vi "Dashboard Main.vi"() -> ()   [LabVIEW 2013]
uses:
  <vilib>/event_ctls.llb/eventvkey.ctl
  <vilib>/Utility/config.llb/NI_LVConfig.lvlib
  <vilib>/Utility/config.llb/Write Key (I32).vi
  <vilib>/Rock Robotics/WPI/Dashboard/WPI_DashboardLogging Global.vi
  <vilib>/Utility/config.llb/Write Key (String).vi
panel:
  out "Image Message":string="Timeout in Camera Communications"
  in  "Rec Mode":enum32{"Stop", "Record", "Playback"}(radio)
  in  "Dashboard Tab":T1(tab)
  out "Left Encoder Distance":dbl
  out "Left Encoder Revolutions":dbl
  out "Left Encoder Agnle":dbl
  out "Right Encoder Distance":dbl
  out "Right Encoder Revolutions":dbl
  out "Right Encoder Agnle":dbl
  out "Slow Drive":bool
  out "Can Shoot":bool
  out "Camera Sonar":dbl
  out "Rear Sonar":dbl
  out "Front Left Sonar":dbl
  out "Front Right Sonar":dbl
  out "Ball in Cannon":bool
  out "Cannon Angle":dbl(knob) scale=0.0..360.0
  out "InTake Angle":dbl(knob) scale=0.0..360.0
  in  "Camera Settings":T2={"Frame Rate"=30, "Compression"=30, "Size"=1} {"Frame Rate" scale=1.0..30.0; "Size" items=["640x480", "320x240", "160x120"]}
  out "MotorSliders R":cluster{"MotorSlide1":dbl, "MotorSlide2":dbl} {"MotorSlide2" scale=-1.0..1.0 scale format="%#_2e"; "MotorSlide1" scale=-1.0..1.0 scale format="%#_2e"}
  out "MotorChart R":cluster{"Numeric":dbl, "Numeric":dbl}(graph)
  out "MotorSliders L":T3 {"MotorSlide4 2" scale=0.0..14.0 scale format="%#_2e"; "MotorSlide2" scale=-1.0..1.0 scale format="%#_2e"; "MotorSlide1" scale=-1.0..1.0 scale format="%#_2e"}
  out "MotorChart L":T4(graph)
  out "JS1 Z":dbl(slide) scale=-1.0..1.0 scale format="%#_2e"
  out "Joystick 1":cluster{"X":dbl, "Y":dbl}[](graph)
  out "JS Buttons 1":T5
  out "JS2 Z":dbl(slide) scale=-1.0..1.0 scale format="%#_2e"
  out "Joystick 2":cluster{"X":dbl, "Y":dbl}[](graph)
  out "JS Buttons 2":T5
  out "Mode":T6(ring)=enum."Auto Disabled"
  out "Camera IP":string
  in  "DB Camera Config":bool
  out "fps":dbl format="%#.1g"
  out "Mbps":dbl format="%#.1g"
  out "Mbps 2":bool
  out "Joystick 3":cluster{"X":dbl, "Y":dbl}[](graph)
  out "JS Buttons 3":T5
  out "JS1 Z 2":dbl(slide) scale=-1.0..1.0 scale format="%#_2e"
  out "Joystick 4":cluster{"X":dbl, "Y":dbl}[](graph)
  out "JS2 Z 2":dbl(slide) scale=-1.0..1.0 scale format="%#_2e"
  out "JS Buttons 4":T5
  in  "Read From Dashboard":bool
  in  "Operator":T7 {"Left Y 2" scale=-1.0..1.0; "Left X 2" scale=-1.0..1.0; "Right Y 2" scale=-1.0..1.0; "Right X 2" scale=-1.0..1.0}
  in  "Drive":T8 {"Left Y" scale=-1.0..1.0; "Left X" scale=-1.0..1.0; "Right Y" scale=-1.0..1.0; "Right X" scale=-1.0..1.0}
  in  "Test Slider":dbl(slide) scale=0.0..100.0 scale format="%#_3g"
  in  "On/Off":bool caption="Solenoid"
  in  "Test Name":u16(ring) items=["Select the test to run...", "Example Test", "-------------------------------", "List of tests is built in robot code.", "Replace with your own automated tests."]
  in  "Test Tree":string(tree)
  in  "Motor":cluster{"Value":dbl, "Enable":bool} {"Value" scale=-1.0..1.0 scale format="%#_3g"}
  out "Progress":T9 {"Test Progress" scale=0.0..100.0}
  in  "Rev/Fwd":cluster{"Forward":bool, "Reverse":bool}
  in  "Test Ring":u16(ring) items=["Auto", "Fixed indoor", "Fixed outdoor 1", "Fixed outdoor 2", "Fixed fluorescent 1", "Fixed fluorescent 2", "Hold current"]
  in  "Listbox":i32(listbox)
  out "Tree":string(tree)
  out "Camera Image":T10(plugin-control)
  in  "Enable":bool
  # "Operation"
  # "Left"
  # "Right"
  # "Left"
  # "Front"
  # "Right"
  # "Battery"
  # "Operation"
  # "Drive"
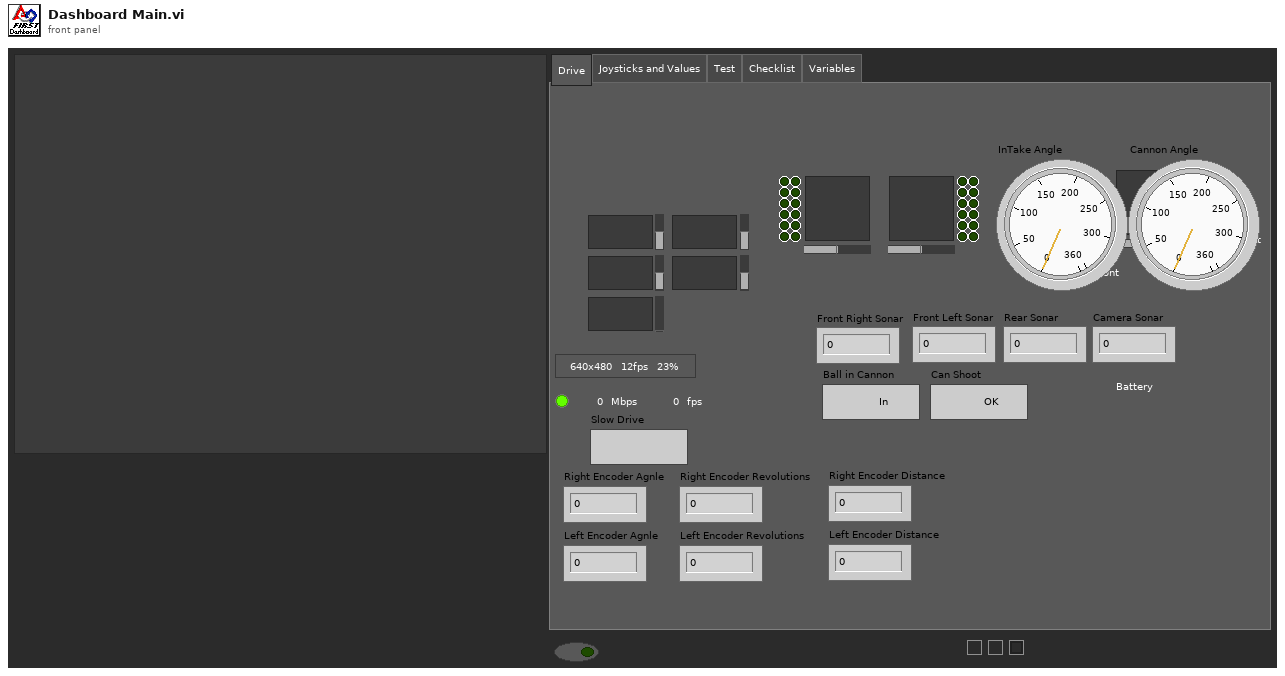
[diagram p1: front panel]
types:
  T1 = enum32{"Drive", "Joysticks and Values", "Test", "Checklist", "Variables"}
  T2 = cluster{"Frame Rate":i32, "Compression":i32, "Size":u16}
  T3 = cluster{"MotorSlide1":dbl, "MotorSlide2":dbl, "MotorSlide4 2":dbl}
  T4 = cluster{"Numeric":dbl, "Numeric":dbl, "Battery":sgl}
  T5 = cluster{bool, bool, bool, bool, bool, bool, bool, bool, bool, bool, bool, bool}
  T6 = enum8{"Tele-Op Disabled", "Tele-Op Enabled", "Auto Disabled", "Auto Enabled", "Test Disabled", "Test Enabled", ""}
  T7 = cluster{"Right X 2":dbl, "Right Y 2":dbl, "Left X 2":dbl, "Left Y 2":dbl, "Arrows 2":dbl, "Left Stick Touch  2":bool, "Right Stick Touch 2":bool, "Left Button  2":bool, "Right Button 2":bool, "L+R Throttles 2":dbl, "Center Right 2":bool, "Center Left 2":bool, "X 2":bool, "A 2":bool, "B 2":bool, "Y 2":bool}
  T8 = cluster{"Right X":dbl, "Right Y":dbl, "Left X":dbl, "Left Y":dbl, "Arrows":dbl, "Left Stick Touch ":bool, "Right Stick Touch":bool, "Left Button ":bool, "Right Button":bool, "L+R Throttles":dbl, "Center Right":bool, "Center Left":bool, "X":bool, "A":bool, "B":bool, "Y":bool}
  T9 = cluster{"Test Progress":u8, "Test Progress Text":string}
  T10 = typedef "IMAQ Image.ctl" = refnum<image>
  T11 = enum32{"Drive", "Operation", "Auto", "Test", "Checklist", "Variables"}
  T12 = typedef "Image Type" = u32
  T13 = cluster{"[0]":void, "[1]":void, "[2]":void, "[3]":void, "[4]":void, "[5]":void, "[6]":void, "[7]":void, "[8]":void}
  T14 = cluster{"Digital Inputs":bool[], "Digital Outputs":bool[]}
  T15 = cluster{"Competition mode":bool, "Robot Link":bool, "Autonomous":bool, "Enabled":bool, "E-Stop":bool, "Simulated":bool, "TestMode":bool, "Docked Window":bool}
  T16 = cluster{"Boolean Array[0]":bool, "Boolean Array[1]":bool, "Boolean Array[2]":bool, "Boolean Array[3]":bool, "Boolean Array[4]":bool, "Boolean Array[5]":bool, "Boolean Array[6]":bool, "Boolean Array[7]":bool, "Boolean Array[8]":bool, "Boolean Array[9]":bool, "Boolean Array[10]":bool, "Boolean Array[11]":bool}
  T17 = typedef "NI_LVConfig.lvlib/Config Data RefNum.ctl" = refnum<k1>
  T18 = typedef "eventvkey.ctl" = enum16{"ASCII", "Enter", "Return", "Shift", "Ctrl", "Alt", "Cmd", "Opt", "Caps", "NumLock", "Clear", "Break", "Up", "Down", "Left", "Right", "Insert", "Delete", "Home", "End", "PageUp", "PageDown", "Escape", "Help", "Pause", "ScrollLock", "F1", "F2", "F3", "F4", "F5", "F6", "F7", "F8", "F9", "F10", "F11", "F12", "F13", "F14", "F15", "F16", "F17", "F18", "F19", "F20", "F21", "F22", "F23", "F24", "Play", "VolumeUp", "VolumeDown", "Mute", "Two Byte Char"}
  T19 = cluster{"Image Size":bool, "Image Type":bool, "Pixel Value":bool, "ROI Information":bool, "Zoom Factor":bool}
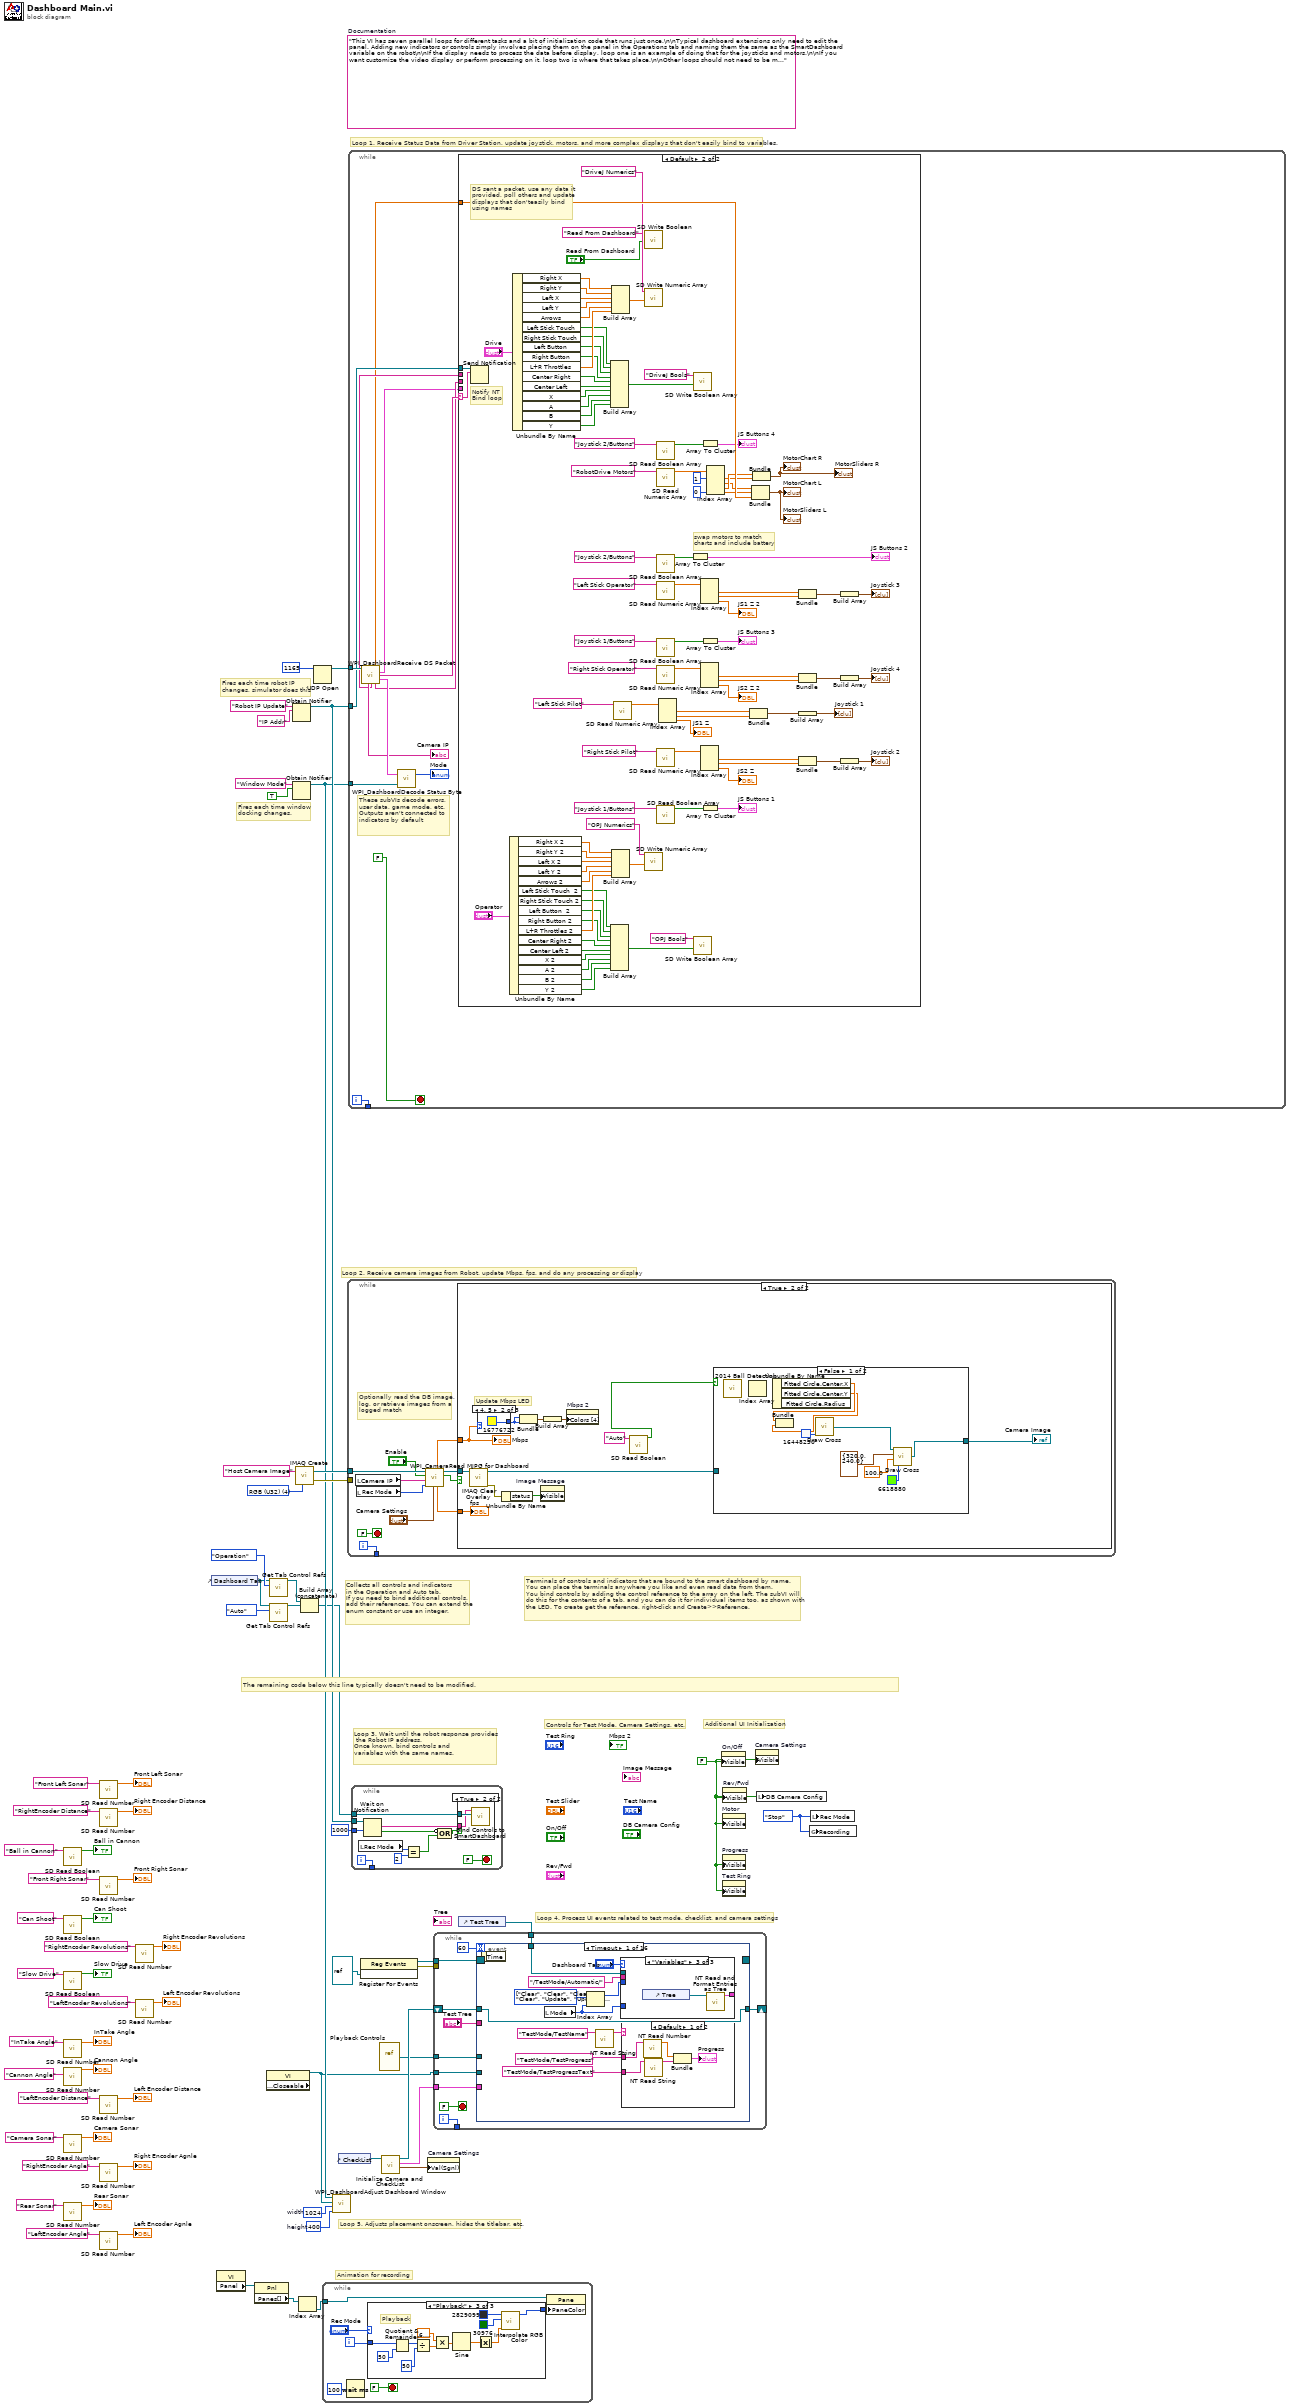
[diagram p0: block diagram]
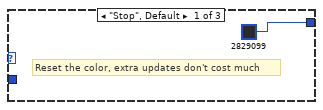
[diagram p2: hidden frame]
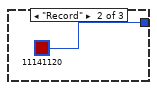
[diagram p3: hidden frame]
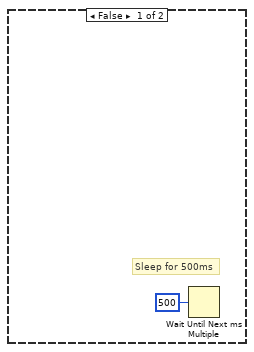
[diagram p5: hidden frame]
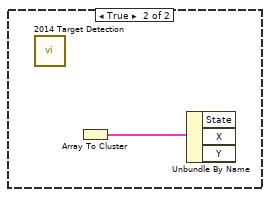
[diagram p6: hidden frame]
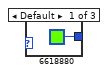
[diagram p7: hidden frame]
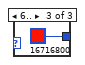
[diagram p8: hidden frame]
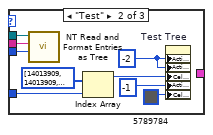
[diagram p10: hidden frame]
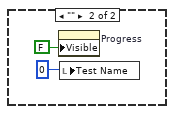
[diagram p11: hidden frame]
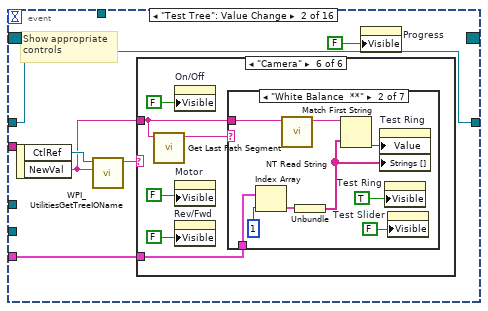
[diagram p12: hidden frame]
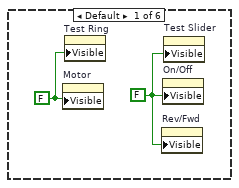
[diagram p13: hidden frame]
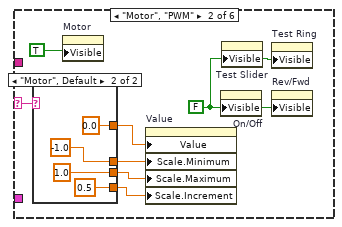
[diagram p14: hidden frame]
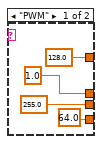
[diagram p15: hidden frame]
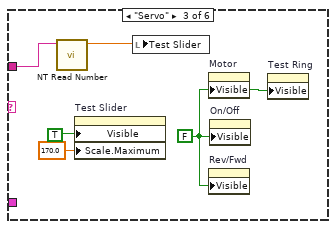
[diagram p16: hidden frame]
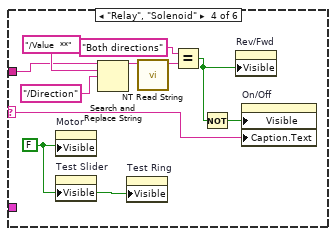
[diagram p17: hidden frame]
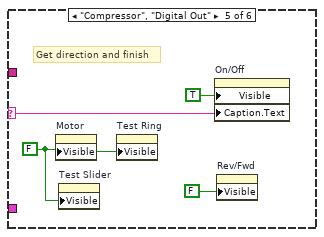
[diagram p18: hidden frame]
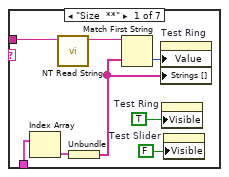
[diagram p19: hidden frame]
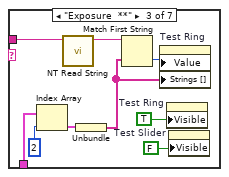
[diagram p20: hidden frame]
diagram:
  w38 = enum32{"Stop", "Record", "Playback"}."Stop" ("Rec Mode")
  w41 = 400  # height
  w42 = 1024  # width
  w55 = FALSE ("Visible")
  (unwired) "This VI has seven parallel loops for different tasks and a bit of initialization code that runs just once.\n\nTypical dashboard extensions only need to edit the panel. Adding new indicators or controls simply involves placing them on the panel in the Operations tab and naming them the same as the SmartDashboard variable on the robot\n\nIf the display needs to process the data before display, loop one is an example of doing that for the joysticks and motors.\n\nIf you want customize the video display or perform processing on it, loop two is where that takes place.\n\nOther loops should not need to be modified. They are pretty standard, and document the task they perform."  # Documentation
  w65 = T12 4 items=["Grayscale (U8)", "Grayscale (I16)", "Grayscale (SGL)", "Complex (CSG)", "RGB (U32)", "HSL (U32)", "RGB (U64)"] ("Image Type")
  # "Controls for Test Mode, Camera Settings, etc."
  # "Additional UI Initialization"
  # "Animation for recording"
  # "Fires each time robot IP\nchanges, simulator does this"
  # "Fires each time window\ndocking changes."
  # "Collects all controls and indicators\nin the Operation and Auto tab.\nIf you need to bind additional controls,\nadd their references. You can extend the\nenum constant or use an integer."
  # "The remaining code below this line typically doesn't need to be modified."
  # "Loop 4. Process UI events related to test mode, checklist, and camera settings"
  # "Terminals of controls and indicators that are bound to the smart dashboard by name.\nYou can place the terminals anywhere you like and even read data from them.\nYou bind controls by adding the control reference to the array on the left. The subVI will\ndo this for the contents of a tab, and you can do it for individual items too, as shown with\nthe LED. To create get the reference, right-click and Create>>Reference."
  # "Loop 3. Wait until the robot response provides\n the Robot IP address.\nOnce known, bind controls and\nvariables with the same names."
  # "Loop 5. Adjusts placement onscreen, hides the titlebar, etc."
  # "Loop 1. Receive Status Data from Driver Station, update joystick, motors, and more complex displays that don't easily bind to variables."
  # "Loop 2. Receive camera images from Robot, update Mbps, fps, and do any processing or display"
  n1 = call <vilib>:"SD Read Boolean.vi"("Name"="Ball in Cannon") -> ("Boolean"=→"Ball in Cannon":bool)  [unwired: 8 in, 2 out]
  n2 = call <vilib>:"SD Read Boolean.vi"("Name"="Can Shoot") -> ("Boolean"=→"Can Shoot":bool)  [unwired: 8 in, 2 out]
  n3 = call <vilib>:"SD Read Boolean.vi"("Name"="Slow Drive") -> ("Boolean"=→"Slow Drive":bool)  [unwired: 8 in, 2 out]
  n4 = call <vilib>:"SD Read Number.vi"("Name"="InTake Angle") -> ("Numeric"=→"InTake Angle":dbl)  [unwired: 8 in, 2 out]
  n5 = call <vilib>:"SD Read Number.vi"("Table Prefix"="Cannon Angle" ("Name")) -> ("Numeric"=→"Cannon Angle":dbl)  [unwired: 8 in, 2 out]
  n6 = call <vilib>:"SD Read Number.vi"("Name"="Camera Sonar") -> ("Numeric"=→"Camera Sonar":dbl)  [unwired: 8 in, 2 out]
  n7 = call <vilib>:"SD Read Number.vi"("Name"="Rear Sonar") -> ("Numeric"=→"Rear Sonar":dbl)  [unwired: 8 in, 2 out]
  n8 = call <vilib>:"SD Read Number.vi"("Name"="Front Left Sonar") -> ("Numeric"=→"Front Left Sonar":dbl)  [unwired: 8 in, 2 out]
  n9 = call <vilib>:"SD Read Number.vi"("Name"="RightEncoder Distance") -> ("Numeric"=→"Right Encoder Distance":dbl)  [unwired: 8 in, 2 out]
  n10 = call <vilib>:"SD Read Number.vi"("Name"="Front Right Sonar") -> ("Numeric"=→"Front Right Sonar":dbl)  [unwired: 8 in, 2 out]
  n11 = call <vilib>:"SD Read Number.vi"("Name"="LeftEncoder Distance") -> ("Numeric"=→"Left Encoder Distance":dbl)  [unwired: 8 in, 2 out]
  n12 = call <vilib>:"SD Read Number.vi"("Name"="RightEncoder Angle") -> ("Numeric"=→"Right Encoder Agnle":dbl)  [unwired: 8 in, 2 out]
  n13 = call <vilib>:"SD Read Number.vi"("Name"="LeftEncoder Angle") -> ("Numeric"=→"Left Encoder Agnle":dbl)  [unwired: 8 in, 2 out]
  n14 = call <vilib>:"SD Read Number.vi"("Name"="RightEncoder Revolutions") -> ("Numeric"=→"Right Encoder Revolutions":dbl)  [unwired: 8 in, 2 out]
  n15 = call <vilib>:"SD Read Number.vi"("Name"="LeftEncoder Revolutions") -> ("Numeric"=→"Left Encoder Revolutions":dbl)  [unwired: 8 in, 2 out]
  n16 = control-ref of="Dashboard Tab"() -> (w36:refnum<vi>)
  n17 = property class="VI"() -> ("Panel"=w49:refnum<vi>)  [unwired: 2 in, 2 out]
  n18 = property class="Pnl"(reference=w49) -> ("Panes[]"=w50:refnum<vi>[])  [unwired: 1 in, 2 out]
  n19 = property class="VI" props=["Front Panel.Closeable"]() -> (reference out=w37:refnum<vi>)  [unwired: 2 in, 2 out]
  n20 = call <vilib>:"Get Tab Control Refs.vi"("Page Index"=T11."Operation" ("Dashboard Tab"), "TabControl in"=w36) -> ("ControlsOnPage"=w34:refnum<vi>[])  [unwired: 9 in]
  n21 = call <vilib>:"Get Tab Control Refs.vi"("Page Index"=T11."Auto" ("Dashboard Tab"), "TabControl in"=w36) -> ("ControlsOnPage"=w35:refnum<vi>[])  [unwired: 9 in]
  n22 = Obtain Notifier(name (unnamed)="Robot IP Update", notification data type="IP Addr" ("name (unnamed)")) -> (notifier out=w59:refnum<notifier>)  [unwired: 2 in, 2 out]
  n23 = Obtain Notifier(name (unnamed)="Window Mode", notification data type=TRUE) -> (notifier out=w40:refnum<notifier>)  [unwired: 2 in, 2 out]
  n24 = call "IMAQ Create"("Image Name"="Host Camera Image", "Image Type"=w65) -> ("New Image"=w63:T10, "error out"=w62:errorcluster)  [unwired: 2 in, 1 out]
  n25 = Index Array(array=w50) -> (element=w48:refnum<vi>)  [unwired: 1 in]
  n26 = Build Array (concatenate)(w34, w35) -> (w33:refnum<vi>[], w31:refnum<vi>[])
  n27 = UDP Open(11:u16 1165 ("port")) -> (port=w66:refnum<k16>)  [unwired: 2 in, 4 out]
  n28 = while {
    tunnel: w48 -> [w69]
    i -> [w72]
    stop <- FALSE stop-if-true
    n29 = Wait (ms)(milliseconds to wait=u32 100) -> ()  [unwired: 1 out]
    n30 = case shown="\"Playback\"" "Rec Mode" {
      tunnel: w72 -> [_ _ w87]
      tunnel: [u32 2829099 ("Base Color") u32 11141120 ("Target Color") w76] -> w68
      frame "Stop", Default {
        # "Reset the color, extra updates don't cost much"
      }
      frame "Record" {
      }
      frame "Playback" {
        # "Playback"
        n31 = Quotient & Remainder(x=w87, y=u32 50 ("milliseconds to wait")) -> (x-y*floor(x/y)=w83:u32)  [unwired: 1 out]
        n32 = Divide(x=w83, y=u32 50 ("milliseconds to wait")) -> (x/y=w80:dbl)
        n33 = Multiply(x=6.283185307179586, y=w80) -> (x*y=w85:dbl)
        n34 = Sine(x=w85) -> (sin(x)=w84:dbl)
        n35 = Absolute Value(x=w84) -> (abs(x)=w77:dbl)
        n36 = call "Interpolate RGB Color.vi"("Proportion"=w77, "Target Color"=u32 30976, "Base Color"=u32 2829099) -> ("Result Color"=w76:u32)  [unwired: 8 in]
      }
    }
    n37 = property class="Pane"(reference=w69, "PaneColor"=w68) -> ()  [unwired: 1 in, 2 out]
  }
  n38 = call <vilib>:"WPI_DashboardAdjust Dashboard Window.vi"("height"=w41, "width"=w42, "reference in"=w37, "Notifier in"=w40) -> ()  [unwired: 8 in]
  n39 = control-ref of="CheckList"() -> (w39:refnum<vi>)
  n40 = while {
    tunnel: w63 -> [w96]
    tunnel: w62 -> [_]
    tunnel: [w97] -> _
    i -> [w97]
    stop <- FALSE stop-if-true
    # "Optionally read the DB image,\nlog, or retrieve images from a\nlogged match"
    n41 = local read "Camera IP"() -> (w89:string)
    n42 = local read "Rec Mode"() -> (w88:enum32{"Stop", "Record", "Playback"})
    n43 = call <vilib>:"WPI_CameraRead MJPG for Dashboard.vi"("Camera Settings"="Camera Settings", "Rec Mode"=w88, "Camera IP"=w89, "Enable"="Enable", "Refnum in"=w96) -> ("Active"=w93:bool, "Refnum out"=w95:T10, "FPS"=w92:dbl, "Bandwidth (Mbps)"=w91:dbl)  [unwired: 3 in]
    n44 = case shown="True" w93 {
      tunnel: w95 -> [_ w106]
      tunnel: w91 -> [_ w105]
      tunnel: w92 -> [_ w104]
      frame False {
        # "Sleep for 500ms"
        n45 = Wait Until Next ms Multiple(millisecond multiple=u32 500) -> ()  [unwired: 1 out]
      }
      frame True {
        # "Update Mbps LED"
        n46 = call "IMAQ Clear Overlay"("Image"=w106) -> ("error out"=w110:errorcluster, "Image Out"=w101:T10)  [unwired: 2 in, 7 out]
        n47 = case shown="4, 5" w105 {
          tunnel: [u32 6618880 ("Color Box") u32 16776722 ("Color Box") u32 16716800 ("Color Box")] -> w107
          frame Default {
          }
          frame 4, 5 {
          }
          frame 6.. {
          }
        }
        n48 = Unbundle By Name(w110) -> ("status"=w111:bool)
        n49 = Bundle("Color Box"=w107, "Color Box"=w107) -> (w109:cluster{"Color Box":u32, "Color Box":u32})  [unwired: 1 out]
        n50 = property on="Image Message" class="Str"("Visible"=w111) -> ()  [unwired: 2 in, 2 out]
        n51 = Build Array(w109) -> (w108:cluster{"Color Box":u32, "Color Box":u32}[])
        n52 = property on="Mbps 2" class="Bool (strict)"("Colors [4]"=w108) -> ()  [unwired: 2 in, 2 out]
        n53 = call <vilib>:"SD Read Boolean.vi"("Name"="Auto") -> ("Boolean"=w102:bool)  [unwired: 8 in, 2 out]
        n54 = case shown="False" w102 {
          tunnel: [w112 _] -> w100
          tunnel: w101 -> [_ _]
          frame False {
            n55 = call "2014 Ball Detection.vi"() -> ()  [unwired: 12 in]
            n56 = Index Array() -> ()  [unwired: 2 in, 1 out]
            n57 = Unbundle By Name() -> ("Fitted Circle.Center.X"=w119:sgl, "Fitted Circle.Center.Y"=w118:sgl)  [unwired: 1 in, 1 out]
            n58 = Bundle("X"=w119, "Y"=w118) -> ()  [unwired: 1 in, 1 out]
            n59 = call "Draw Cross.vi"("Color"=u32 16448250) -> ("Image Out"=w116:T10)  [unwired: 3 in]
            n60 = call "Draw Cross.vi"("Color"=u32 6618880, "Cross Size"=100.0, "Cluster"=cluster{"Center X":dbl, "Center Y":dbl} {"Center X"=320.0, "Center Y"=240.0}, "Image"=w116) -> ("Image Out"=w112:T10)
          }
          frame True {
            n61 = call "2014 Target Detection.vi"() -> ()  [unwired: 12 in]
            n62 = Array To Cluster() -> (cluster=w120:T13)  [unwired: 1 in]
            n63 = Unbundle By Name(w120) -> ()  [unwired: 3 out]
          }
        }
        "Camera Image" <- w100
        "Mbps" <- w105
        "fps" <- w104
      }
    }
  }
  n64 = while {
    tunnel: w66 -> [w134]
    tunnel: w59 -> [w129]
    tunnel: w40 -> [w133]
    tunnel: [w130] -> _
    i -> [w130]
    stop <- FALSE stop-if-true
    # "These subVIs decode errors, user data, game mode, etc.\nOutputs aren't connected to indicators by default"
    n65 = call <vilib>:"WPI_DashboardReceive DS Packet.vi"("Recv Socket"=w134) -> ("Battery"=w124:sgl, "Driver Station"=w125:T14, "Robot IP Address"=w128:string, "Status"=w135:T15, "Camera IP Address"=→"Camera IP":string, "Low Priority User Data"=w127:string, "High Priority User Data"=w126:string)  [unwired: 1 in, 7 out]
    n66 = call <vilib>:"WPI_DashboardDecode Status Byte.vi"("Window Mode Notifier"=w133, "Status"=w135) -> ("Mode"=→"Mode":T6)  [unwired: 1 out]
    n67 = case shown="Default" w128 {
      selector: w128 -> [_ w211]
      tunnel: w129 -> [_ w212]
      tunnel: w127 -> [_ _]
      tunnel: w126 -> [_ _]
      tunnel: w125 -> [_ _]
      tunnel: w124 -> [_ w210]
      frame "0.0.0.0" {
        # "DS not sending packets, or no robot exists yet.\nDon't poll the variables"
      }
      frame Default {
        # "Notify NT\nBind loop"
        # "DS sent a packet. use any data it\nprovided, poll others and update\ndisplays that don'teasily bind\nusing names"
        # "swap motors to match\ncharts and include battery"
        n68 = Send Notification(notification=w211, notifier=w212) -> ()  [unwired: 1 in, 2 out]
        n69 = Unbundle By Name("Operator") -> ("Right X 2"=w156:dbl, "Right Y 2"=w155:dbl, "Left X 2"=w154:dbl, "Left Y 2"=w153:dbl, "Arrows 2"=w152:dbl, "Left Stick Touch  2"=w150:bool, "Right Stick Touch 2"=w149:bool, "Left Button  2"=w148:bool, "Right Button 2"=w147:bool, "L+R Throttles 2"=w151:dbl, "Center Right 2"=w146:bool, "Center Left 2"=w145:bool, "X 2"=w144:bool, "A 2"=w143:bool, "B 2"=w142:bool, "Y 2"=w141:bool)
        n70 = Unbundle By Name("Drive") -> ("Right X"=w177:dbl, "Right Y"=w176:dbl, "Left X"=w175:dbl, "Left Y"=w174:dbl, "Arrows"=w173:dbl, "Left Stick Touch"=w170:bool, "Right Stick Touch"=w169:bool, "Left Button"=w168:bool, "Right Button"=w167:bool, "L+R Throttles"=w172:dbl, "Center Right"=w165:bool, "Center Left"=w164:bool, "X"=w163:bool, "A"=w162:bool, "B"=w161:bool, "Y"=w160:bool)
        n71 = Build Array(w170, w169, w168, w167, w165, w164, w163, w162, w161, w160) -> (w166:bool[])
        n72 = Build Array(w150, w149, w148, w147, w146, w145, w144, w143, w142, w141) -> (w159:bool[])
        n73 = Build Array(w177, w176, w175, w174, w173, w172) -> (w178:dbl[])
        n74 = Build Array(w156, w155, w154, w153, w152, w151) -> (w137:dbl[])
        n75 = call <vilib>:"SD Read Numeric Array.vi"("Name"="Left Stick Pilot") -> ("Numeric Array"=w228:dbl[])  [unwired: 8 in, 2 out]
        n76 = call <vilib>:"SD Write Boolean.vi"("Boolean"="Read From Dashboard", "Name"="Read From Dashboard") -> ()  [unwired: 8 in, 2 out]
        n77 = call <vilib>:"SD Write Numeric Array.vi"("Numeric Array"=w178, "Name"="DriveJ Numerics") -> ()  [unwired: 8 in, 2 out]
        n78 = call <vilib>:"SD Write Numeric Array.vi"("Numeric Array"=w137, "Name"="OPJ Numerics") -> ()  [unwired: 8 in, 2 out]
        n79 = call <vilib>:"SD Read Boolean Array.vi"("Name"="Joystick 2/Buttons") -> ("Boolean Array"=w190:bool[])  [unwired: 8 in, 2 out]
        n80 = call <vilib>:"SD Read Numeric Array.vi"("Name"="RobotDrive Motors") -> ("Numeric Array"=w209:dbl[])  [unwired: 8 in, 2 out]
        n81 = call <vilib>:"SD Read Boolean Array.vi"("Name"="Joystick 2/Buttons") -> ("Boolean Array"=w221:bool[])  [unwired: 8 in, 2 out]
        n82 = call <vilib>:"SD Read Numeric Array.vi"("Name"="Left Stick Operator") -> ("Numeric Array"=w197:dbl[])  [unwired: 8 in, 2 out]
        n83 = call <vilib>:"SD Read Boolean Array.vi"("Name"="Joystick 1/Buttons") -> ("Boolean Array"=w199:bool[])  [unwired: 8 in, 2 out]
        n84 = call <vilib>:"SD Read Numeric Array.vi"("Name"="Right Stick Operator") -> ("Numeric Array"=w191:dbl[])  [unwired: 8 in, 2 out]
        n85 = call <vilib>:"SD Read Numeric Array.vi"("Name"="Right Stick Pilot") -> ("Numeric Array"=w222:dbl[])  [unwired: 8 in, 2 out]
        n86 = call <vilib>:"SD Read Boolean Array.vi"("Name"="Joystick 1/Buttons") -> ("Boolean Array"=w230:bool[])  [unwired: 8 in, 2 out]
        n87 = Index Array(array=w228) -> (element #1=w225:dbl, element #2=w226:dbl, element #3=→"JS1 Z":dbl)  [unwired: 3 in]
        n88 = Array To Cluster(array=w221) -> (cluster=→"JS Buttons 2":T16)
        n89 = call <vilib>:"SD Write Boolean Array.vi"("Boolean Array"=w166, "Name"="DriveJ Bools") -> ()  [unwired: 8 in, 2 out]
        n90 = call <vilib>:"SD Write Boolean Array.vi"("Boolean Array"=w159, "Name"="OPJ Bools") -> ()  [unwired: 8 in, 2 out]
        n91 = Index Array(array=w197) -> (element #1=w194:dbl, element #2=w195:dbl, element #3=→"JS1 Z 2":dbl)  [unwired: 3 in]
        n92 = Index Array(array=w191) -> (element #1=w187:dbl, element #2=w186:dbl, element #3=→"JS2 Z 2":dbl)  [unwired: 3 in]
        n93 = Index Array(array=w222) -> (element #1=w217:dbl, element #2=w216:dbl, element #3=→"JS2 Z":dbl)  [unwired: 3 in]
        n94 = Array To Cluster(array=w190) -> (cluster=→"JS Buttons 4":T16)
        n95 = Array To Cluster(array=w199) -> (cluster=→"JS Buttons 3":T16)
        n96 = Array To Cluster(array=w230) -> (cluster=→"JS Buttons 1":T16)
        n97 = Index Array(array=w209, index #1=1, index #4=0) -> (element #1=w205:dbl, element #2=w204:dbl, element #3=w206:dbl, element #4=w201:dbl)  [unwired: 2 in]
        n98 = Bundle("Numeric"=w225, "Numeric"=w226) -> (w224:cluster{"Numeric":dbl, "Numeric":dbl})  [unwired: 1 in]
        n99 = Bundle("Numeric"=w204, "Numeric"=w201, "Battery"=w210) -> (→"MotorChart L" →"MotorSliders L":T4)  [unwired: 1 in]
        n100 = Bundle("Numeric"=w206, "Numeric"=w205) -> (→"MotorChart R" →"MotorSliders R":cluster{"Numeric":dbl, "Numeric":dbl})  [unwired: 1 in]
        n101 = Build Array(w224) -> (→"Joystick 1":cluster{"Numeric":dbl, "Numeric":dbl}[])
        n102 = Bundle("Numeric"=w194, "Numeric"=w195) -> (w193:cluster{"Numeric":dbl, "Numeric":dbl})  [unwired: 1 in]
        n103 = Bundle("Numeric"=w187, "Numeric"=w186) -> (w188:cluster{"Numeric":dbl, "Numeric":dbl})  [unwired: 1 in]
        n104 = Bundle("Numeric"=w217, "Numeric"=w216) -> (w218:cluster{"Numeric":dbl, "Numeric":dbl})  [unwired: 1 in]
        n105 = Build Array(w193) -> (→"Joystick 3":cluster{"Numeric":dbl, "Numeric":dbl}[])
        n106 = Build Array(w188) -> (→"Joystick 4":cluster{"Numeric":dbl, "Numeric":dbl}[])
        n107 = Build Array(w218) -> (→"Joystick 2":cluster{"Numeric":dbl, "Numeric":dbl}[])
      }
    }
  }
  n108 = while {
    tunnel: w33 -> [w244]
    tunnel: w59 -> [w242]
    tunnel: [w240] -> _
    tunnel: u32 1000 ("milliseconds to wait") -> [w239]
    i -> [w240]
    stop <- FALSE stop-if-true
    n109 = local read "Rec Mode"() -> (w235:enum32{"Stop", "Record", "Playback"})
    n110 = Wait on Notification(notifier=w242, timeout in ms (-1)=w239) -> (notification=w241:string, timed out?=w237:bool)  [unwired: 2 in, 2 out]
    n111 = Equal?(x=w235, y=u16 2 ("Rec Mode")) -> (x = y?=w236:bool)
    n112 = Compound Arithmetic op=OR(invert w237, w236) -> (w238:bool)
    n113 = case shown="True" w238 {
      tunnel: w244 -> [_ w246]
      tunnel: w241 -> [_ w245]
      frame False {
      }
      frame True {
        n114 = call <vilib>:"Bind Controls to SmartDashboard.vi"("Bound Control Refs"=w246, "Server IP Address"=w245) -> ()  [unwired: 10 in]
      }
    }
  }
  n115 = register-events(refnum<vi> refnum) -> (reference out=w46:refnum<event-registration>, error out=w45:errorcluster)  [unwired: 2 in]
  n116 = vi-ref "Playback Controls.vi"() -> (w47:refnum<vi>)
  n117 = call "Initialize Camera and CheckList.vi"("ListBox in"=w39) -> ("Cluster"=w53:cluster{"value":i32, "value":i32, "index":i32}, "Array"=w54:cluster{string[]}[], "File Refnum"=w52:T17)  [unwired: 8 in]
  n118 = property on="Camera Settings" class="Clust (strict)"("Val(Sgnl)"=w53) -> ()  [unwired: 2 in, 2 out]
  n119 = control-ref of="Test Tree"() -> (w51:refnum<vi>)
  n120 = while {
    tunnel: w54 -> [w254]
    shift-right: [w253] -> _
    shift-left: w52 -> [w252]
    tunnel: [w251] -> _
    tunnel: w51 -> [w250]
    tunnel: w47 -> [w249]
    tunnel: w46 -> [w248]
    tunnel: w45 -> [_]
    tunnel: w37 -> [w247]
    i -> [w251]
    stop <- FALSE stop-if-true
    n121 = event shown="[0] Timeout" {
      selector: w248 -> [_ _ _ _ _ _ _ _ _ _ _ _ _ _ _ _]
      dyn-events: [_ _ _ _ _ _ _ _ _ _ _ _ _ w492 _ _] -> _
      timeout: u32 60 ("milliseconds to wait") -> [_ _ _ _ _ _ _ _ _ _ _ _ _ _ _ _]
      tunnel: w250 -> [w264 _ _ _ _ _ _ _ _ _ _ _ _ _ _ _]
      tunnel: "Test Tree" -> [_ _ _ _ _ _ _ _ w461 w469 w471 w475 w483 _ _ _]
      tunnel: w254 -> [_ w288 _ _ _ _ w425 w455 _ _ _ _ _ _ _ _]
      tunnel: [w258 w287 w386 w391 w399 w411 w424 w448 w460 w467 w470 w474 w482 w494 w508 w509] -> w253
      tunnel: w252 -> [w258 w287 w386 w391 w399 w411 w423 w448 w460 w467 w470 w474 w482 w494 w508 w509]
      tunnel: w249 -> [_ _ _ _ _ _ _ _ _ _ _ _ _ w495 _ w512]
      tunnel: w247 -> [_ _ _ _ _ _ _ _ _ _ _ _ _ w490 _ _]
      event Timeout {
        w263 = enum16{"Update", "Clear"}[] [enum."Clear", enum."Clear", enum."Clear", enum."Clear", enum."Update", enum."Update", enum."Clear"] items=["Update", "Clear"]
        n122 = event-data() -> ()  [unwired: 1 in, 1 out]
        n123 = local read "Mode"() -> (w261:T6)
        n124 = Index Array(array=w263, index=w261) -> (element=w262:enum16{"Update", "Clear"})
        n125 = call <vilib>:"NT Read String.vi"("Name"="TestMode/TestName") -> ("String"=w267:string)  [unwired: 9 in, 1 out]
        n126 = case shown="\"Variables\"" "Dashboard Tab" {
          tunnel: w264 -> [_ w277 _]
          tunnel: "/TestMode/Automatic/" ("Name Pattern") -> [_ w276 _]
          tunnel: w262 -> [_ w275 _]
          tunnel: w261 -> [_ w273 _]
          tunnel: [_ _ w279] -> _
          frame "Test", Default {
          }
          frame "Test" {
            w272 = -2 ("Active Item:Row Number")
            n127 = call <vilib>:"NT Read and Format Entries as Tree.vi"("Operation"=w275, "Name Pattern"=w276, "Tree Refnum"=w277) -> ()  [unwired: 7 in, 2 out]
            n128 = Index Array(array=u32[] [14013909, 14013909, 14013909, 14013909, 14013909, 16777215, 14013909], index=w273) -> (element=w271:u32)
            n129 = property on="Test Tree" class="Tree (strict)"("Active Item Row Number"=w272, "ActiveColNum"=w272, "CellBG"=w271, "Active Item Row Number"=-1 ("Active Item:Row Number"), "CellBG"=u32 5789784 ("Color Box")) -> ()  [unwired: 2 in, 2 out]
          }
          frame "Variables" {
            n130 = control-ref of="Tree"() -> (w278:refnum<vi>)
            n131 = call <vilib>:"NT Read and Format Entries as Tree.vi"("Tree Refnum"=w278) -> ("Formatted Strings"=w279:cluster{"Name":string, "Value":string}[])  [unwired: 9 in, 1 out]
          }
        }
        n132 = case shown="Default" w267 {
          tunnel: "TestMode/TestProgress" ("Name") -> [w281 _]
          tunnel: "TestMode/TestProgressText" ("Name") -> [w280 _]
          frame Default {
            n133 = call <vilib>:"NT Read Number.vi"("Name"=w281) -> ("Numeric"=w282:dbl)  [unwired: 9 in, 1 out]
            n134 = call <vilib>:"NT Read String.vi"("Name"=w280) -> ("String"=w283:string)  [unwired: 9 in, 1 out]
            n135 = Bundle("Numeric"=w282, "String"=w283) -> (→"Progress":cluster{"Numeric":dbl, "String":string})  [unwired: 1 in]
          }
          frame "" {
            n136 = property on="Progress" class="Clust (strict)"("Visible"=FALSE) -> ()  [unwired: 2 in, 2 out]
            n137 = local write "Test Name"(u16 0) -> ()
          }
        }
      }
      event "Test Tree": Value Change {
        # "Show appropriate\ncontrols"
        n138 = event-data() -> ("CtlRef"=w291:refnum<vi>, "NewVal"=w289:string)  [unwired: 1 in]
        n139 = call <vilib>:"WPI_UtilitiesGetTreeIOName.vi"("NewVal"=w289, "TreeControl in"=w291) -> ("I/O Name"=w292:string)  [unwired: 9 in]
        n140 = case shown="\"Camera\"" w292 {
          selector: w292 -> [_ w299 _ w317 w326 _]
          tunnel: w289 -> [_ _ w314 w316 _ w333]
          tunnel: w288 -> [_ _ _ _ _ w332]
          frame Default {
            w294 = FALSE ("Visible")
            w293 = FALSE ("Visible")
            n141 = property on="Motor" class="Clust (strict)"("Visible"=w293) -> ()  [unwired: 2 in, 2 out]
            n142 = property on="Test Ring" class="Ring (strict)"("Visible"=w293) -> ()  [unwired: 2 in, 2 out]
            n143 = property on="Rev/Fwd" class="Clust (strict)"("Visible"=w294) -> ()  [unwired: 2 in, 2 out]
            n144 = property on="On/Off" class="Bool (strict)"("Visible"=w294) -> ()  [unwired: 2 in, 2 out]
            n145 = property on="Test Slider" class="Slide (strict)"("Visible"=w294) -> ()  [unwired: 2 in, 2 out]
          }
          frame "Motor", "PWM" {
            w300 = FALSE ("Visible")
            n146 = case shown="\"Motor\", Default" w299 {
              tunnel: [1.0 ("Value") -1.0 ("Value")] -> w298
              tunnel: [255.0 ("Value") 1.0 ("Value")] -> w297
              tunnel: [128.0 ("Value") 0.0 ("Value")] -> w296
              tunnel: [64.0 ("Value") 0.5 ("Value")] -> w295
              frame "PWM" {
              }
              frame "Motor", Default {
              }
            }
            n147 = property on="Motor" class="Clust (strict)"("Visible"=TRUE) -> ()  [unwired: 2 in, 2 out]
            n148 = property on="Value" class="Slide (strict)"("Value"=w296, "Scale.Minimum"=w298, "Scale.Maximum"=w297, "Scale.Increment"=w295) -> ()  [unwired: 2 in, 2 out]
            n149 = property on="On/Off" class="Bool (strict)"("Visible"=w300) -> ()  [unwired: 2 in, 2 out]
            n150 = property on="Test Slider" class="Slide (strict)"("Visible"=w300) -> ()  [unwired: 2 in, 2 out]
            n151 = property on="Test Ring" class="Ring (strict)"("Visible"=w300) -> ()  [unwired: 2 in, 2 out]
            n152 = property on="Rev/Fwd" class="Clust (strict)"("Visible"=w300) -> ()  [unwired: 2 in, 2 out]
          }
          frame "Servo" {
            w312 = FALSE ("Visible")
            n153 = call <vilib>:"NT Read Number.vi"("Name"=w314) -> ("Numeric"=w313:dbl)  [unwired: 9 in, 1 out]
            n154 = property on="Test Slider" class="Slide (strict)"("Visible"=TRUE, "Scale.Maximum"=170.0 ("Scale.Range:Maximum")) -> ()  [unwired: 2 in, 2 out]
            n155 = local write "Test Slider"(w313) -> ()
            n156 = property on="Motor" class="Clust (strict)"("Visible"=w312) -> ()  [unwired: 2 in, 2 out]
            n157 = property on="Rev/Fwd" class="Clust (strict)"("Visible"=w312) -> ()  [unwired: 2 in, 2 out]
            n158 = property on="On/Off" class="Bool (strict)"("Visible"=w312) -> ()  [unwired: 2 in, 2 out]
            n159 = property on="Test Ring" class="Ring (strict)"("Visible"=w312) -> ()  [unwired: 2 in, 2 out]
          }
          frame "Relay", "Solenoid" {
            w315 = FALSE ("Visible")
            n160 = property on="Motor" class="Clust (strict)"("Visible"=w315) -> ()  [unwired: 2 in, 2 out]
            n161 = property on="Test Slider" class="Slide (strict)"("Visible"=w315) -> ()  [unwired: 2 in, 2 out]
            n162 = Search and Replace String(input string=w316, search string="/Value  **", replace string="/Direction") -> (result string=w322:string)  [unwired: 5 in, 3 out]
            n163 = property on="Test Ring" class="Ring (strict)"("Visible"=w315) -> ()  [unwired: 2 in, 2 out]
            n164 = call <vilib>:"NT Read String.vi"("Name"=w322) -> ("String"=w320:string)  [unwired: 9 in, 1 out]
            n165 = Equal?(x="Both directions", y=w320) -> (x = y?=w318:bool)
            n166 = Not(x=w318) -> (.not. x?=w319:bool)
            n167 = property on="Rev/Fwd" class="Clust (strict)"("Visible"=w318) -> ()  [unwired: 2 in, 2 out]
            n168 = property on="On/Off" class="Bool (strict)"("Visible"=w319, "Caption.Text"=w317) -> ()  [unwired: 2 in, 2 out]
          }
          frame "Compressor", "Digital Out" {
            w325 = FALSE ("Visible")
            # "Get direction and finish"
            n169 = property on="Motor" class="Clust (strict)"("Visible"=w325) -> ()  [unwired: 2 in, 2 out]
            n170 = property on="Test Slider" class="Slide (strict)"("Visible"=w325) -> ()  [unwired: 2 in, 2 out]
            n171 = property on="Test Ring" class="Ring (strict)"("Visible"=w325) -> ()  [unwired: 2 in, 2 out]
            n172 = property on="On/Off" class="Bool (strict)"("Visible"=TRUE, "Caption.Text"=w326) -> ()  [unwired: 2 in, 2 out]
            n173 = property on="Rev/Fwd" class="Clust (strict)"("Visible"=FALSE) -> ()  [unwired: 2 in, 2 out]
          }
          frame "Camera" {
            n174 = call <vilib>:"Get Last Path Segment.vi"("String in"=w333) -> ("String out"=w334:string)  [unwired: 10 in]
            n175 = property on="On/Off" class="Bool (strict)"("Visible"=FALSE) -> ()  [unwired: 2 in, 2 out]
            n176 = property on="Motor" class="Clust (strict)"("Visible"=FALSE) -> ()  [unwired: 2 in, 2 out]
            n177 = property on="Rev/Fwd" class="Clust (strict)"("Visible"=FALSE) -> ()  [unwired: 2 in, 2 out]
            n178 = case shown="\"White Balance  **\"" w334 {
              tunnel: w333 -> [w340 w349 w358 w367 w376 _ w382]
              tunnel: w332 -> [w338 w346 w355 w364 w373 _ _]
              frame "Size  **" {
                n179 = Index Array(array=w338) -> (element=w337:cluster{string[]})  [unwired: 1 in]
                n180 = call <vilib>:"NT Read String.vi"("Name"=w340) -> ("String"=w339:string)  [unwired: 9 in, 1 out]
                n181 = Unbundle(w337) -> (w335:string[])
                n182 = Match First String(2:w335, 3:w339) -> (0:w336:i32)  [unwired: 1 out]
                n183 = property on="Test Ring" class="Ring (strict)"("Value"=w336, "Strings []"=w335) -> ()  [unwired: 2 in, 2 out]
                n184 = property on="Test Ring" class="Ring (strict)"("Visible"=TRUE) -> ()  [unwired: 2 in, 2 out]
                n185 = property on="Test Slider" class="Slide (strict)"("Visible"=FALSE) -> ()  [unwired: 2 in, 2 out]
              }
              frame "White Balance  **" {
                n186 = Index Array(array=w346, index=1) -> (element=w347:cluster{string[]})
                n187 = call <vilib>:"NT Read String.vi"("Name"=w349) -> ("String"=w348:string)  [unwired: 9 in, 1 out]
                n188 = Unbundle(w347) -> (w344:string[])
                n189 = Match First String(2:w344, 3:w348) -> (0:w343:i32)  [unwired: 1 out]
                n190 = property on="Test Ring" class="Ring (strict)"("Value"=w343, "Strings []"=w344) -> ()  [unwired: 2 in, 2 out]
                n191 = property on="Test Ring" class="Ring (strict)"("Visible"=TRUE) -> ()  [unwired: 2 in, 2 out]
                n192 = property on="Test Slider" class="Slide (strict)"("Visible"=FALSE) -> ()  [unwired: 2 in, 2 out]
              }
              frame "Exposure  **" {
                n193 = Index Array(array=w355, index=2) -> (element=w356:cluster{string[]})
                n194 = call <vilib>:"NT Read String.vi"("Name"=w358) -> ("String"=w357:string)  [unwired: 9 in, 1 out]
                n195 = Unbundle(w356) -> (w352:string[])
                n196 = Match First String(2:w352, 3:w357) -> (0:w353:i32)  [unwired: 1 out]
                n197 = property on="Test Ring" class="Ring (strict)"("Value"=w353, "Strings []"=w352) -> ()  [unwired: 2 in, 2 out]
                n198 = property on="Test Ring" class="Ring (strict)"("Visible"=TRUE) -> ()  [unwired: 2 in, 2 out]
                n199 = property on="Test Slider" class="Slide (strict)"("Visible"=FALSE) -> ()  [unwired: 2 in, 2 out]
              }
              frame "Exposure Priority  **" {
                n200 = Index Array(array=w364, index=3) -> (element=w365:cluster{string[]})
                n201 = call <vilib>:"NT Read String.vi"("Name"=w367) -> ("String"=w366:string)  [unwired: 9 in, 1 out]
                n202 = Unbundle(w365) -> (w361:string[])
                n203 = Match First String(2:w361, 3:w366) -> (0:w362:i32)  [unwired: 1 out]
                n204 = property on="Test Ring" class="Ring (strict)"("Value"=w362, "Strings []"=w361) -> ()  [unwired: 2 in, 2 out]
                n205 = property on="Test Ring" class="Ring (strict)"("Visible"=TRUE) -> ()  [unwired: 2 in, 2 out]
                n206 = property on="Test Slider" class="Slide (strict)"("Visible"=FALSE) -> ()  [unwired: 2 in, 2 out]
              }
              frame "Color Enable  **" {
                n207 = Index Array(array=w373, index=4) -> (element=w374:cluster{string[]})
                n208 = call <vilib>:"NT Read String.vi"("Name"=w376) -> ("String"=w375:string)  [unwired: 9 in, 1 out]
                n209 = Unbundle(w374) -> (w370:string[])
                n210 = Match First String(2:w370, 3:w375) -> (0:w371:i32)  [unwired: 1 out]
                n211 = property on="Test Ring" class="Ring (strict)"("Value"=w371, "Strings []"=w370) -> ()  [unwired: 2 in, 2 out]
                n212 = property on="Test Ring" class="Ring (strict)"("Visible"=TRUE) -> ()  [unwired: 2 in, 2 out]
                n213 = property on="Test Slider" class="Slide (strict)"("Visible"=FALSE) -> ()  [unwired: 2 in, 2 out]
              }
              frame Default {
                n214 = property on="Test Ring" class="Ring (strict)"("Visible"=FALSE) -> ()  [unwired: 2 in, 2 out]
                n215 = property on="Test Slider" class="Slide (strict)"("Visible"=FALSE) -> ()  [unwired: 2 in, 2 out]
              }
              frame "Brightness  **", "Color Level  **", "Compression  **", "FPS  **", "Sharpness  **" {
                n216 = call <vilib>:"NT Read Number.vi"("Name"=w382) -> ("Numeric"=w381:dbl)  [unwired: 9 in, 1 out]
                n217 = local write "Test Slider"(w381) -> ()
                n218 = property on="Test Slider" class="Slide (strict)"("Visible"=TRUE, "Scale.Maximum"=100.0 ("Scale.Range:Maximum")) -> ()  [unwired: 2 in, 2 out]
                n219 = property on="Test Ring" class="Ring (strict)"("Visible"=FALSE) -> ()  [unwired: 2 in, 2 out]
              }
            }
          }
        }
        n220 = property on="Progress" class="Clust (strict)"("Visible"=FALSE) -> ()  [unwired: 2 in, 2 out]
      }
      event "Test Name": Mouse Enter {
        # "Populate the ring with the list of tests"
        n221 = event-data() -> ()  [unwired: 1 in, 1 out]
        n222 = call <vilib>:"NT Read String Array.vi"("Name"="TestMode/TestList") -> ("String Array"=w390:string[])  [unwired: 9 in, 1 out]
        n223 = Build Array (concatenate)("Select the test to run...", w390) -> (w389:string[])
        n224 = property on="Test Name" class="Ring (strict)"("Strings []"=w389) -> ()  [unwired: 2 in, 2 out]
      }
      event "Test Name": Value Change {
        w392 = FALSE ("Visible")
        # "Tell the robot the test name to run"
        n225 = event-data() -> ("NewVal"=w396:u16)  [unwired: 1 in]
        n226 = property on="Test Name" class="Ring (strict)"() -> ("Strings []"=w397:string[])  [unwired: 2 in, 2 out]
        n227 = local write "Progress"(T9 {"Test Progress"=0, "Test Progress Text"=""} ("Progress")) -> ()
        n228 = Index Array(array=w397, index=w396) -> (element=w395:string)
        n229 = call <vilib>:"NT Write String.vi"("String"=w395, "Name"="TestMode/TestName") -> ()  [unwired: 9 in, 1 out]
        n230 = property on="Progress" class="Clust (strict)"("Visible"=TRUE) -> ()  [unwired: 2 in, 2 out]
        n231 = property on="Motor" class="Clust (strict)"("Visible"=w392) -> ()  [unwired: 2 in, 2 out]
        n232 = property on="Test Slider" class="Slide (strict)"("Visible"=w392) -> ()  [unwired: 2 in, 2 out]
        n233 = property on="On/Off" class="Bool (strict)"("Visible"=w392) -> ()  [unwired: 2 in, 2 out]
        n234 = property on="Rev/Fwd" class="Clust (strict)"("Visible"=w392) -> ()  [unwired: 2 in, 2 out]
        n235 = property on="Test Ring" class="Ring (strict)"("Visible"=w392) -> ()  [unwired: 2 in, 2 out]
      }
      event "Listbox": Double Click {
        n236 = event-data() -> ("PlatMods.Shift"=w400:bool, "Row"=w402:i32)  [unwired: 1 in]
        n237 = case shown="True" w400 {
          tunnel: w402 -> [w406 _]
          tunnel: 1 -> [w405 _]
          frame False {
            n238 = property on="Listbox" class="LstBox (strict)"() -> ("Item Symbols"=w404:i32[])  [unwired: 2 in, 2 out]
            n239 = Replace Array Subset(array=w404, new element=w405, index=w406) -> (w403:i32[])
            n240 = property on="Listbox" class="LstBox (strict)"("Item Symbols"=w403) -> ()  [unwired: 2 in, 2 out]
          }
          frame True {
            w407 = 0 ("Top Row")
            n241 = property on="Listbox" class="LstBox (strict)"() -> ("Number of Rows"=w409:u32)  [unwired: 2 in, 2 out]
            n242 = Initialize Array(0, w409) -> (w408:i32[])
            n243 = property on="Listbox" class="LstBox (strict)"("Top Row"=w407, "Value"=w407, "Item Symbols"=w408) -> ()  [unwired: 2 in, 2 out]
          }
        }
      }
      event "Listbox": Key Down {
        n244 = event-data() -> ("VKey"=w413:T18)  [unwired: 1 in]
        n245 = case shown="\"Left\", \"Right\"" w413 {
          selector: w413 -> [w418 _]
          tunnel: eventvkey."Left" ("VKey") -> [w416 _]
          frame "Left", "Right" {
            n246 = Equal?(x=w416, y=w418) -> (x = y?=w417:bool)
            n247 = Select(t=0, s=w417, f=1) -> (s? t:f=w419:i32)
            n248 = property on="Listbox" class="LstBox (strict)"() -> ("Item Symbols"=w422:i32[])  [unwired: 2 in, 2 out]
            n249 = Replace Array Subset(array=w422, new element=w419, index="Listbox") -> (w421:i32[])
            n250 = property on="Listbox" class="LstBox (strict)"("Item Symbols"=w421) -> ()  [unwired: 2 in, 2 out]
          }
          frame Default {
          }
        }
      }
      event "DB Camera Config": Value Change {
        n251 = event-data() -> ("NewVal"=w426:bool)  [unwired: 1 in]
        n252 = case shown="False" w426 {
          tunnel: w425 -> [w435 _]
          tunnel: [w428 w446] -> w424
          tunnel: w423 -> [w427 w446]
          frame False {
            w442 = "Camera"
            w445 = FALSE ("Visible")
            n253 = local read "Camera Settings"() -> (w434:T2)
            n254 = Index Array(array=w435) -> (element=w438:cluster{string[]})  [unwired: 1 in]
            n255 = Unbundle(w434) -> ("Frame Rate"=w433:i32, "Compression"=w432:i32, "Size"=w436:u16)
            n256 = Unbundle(w438) -> (w437:string[])
            n257 = Index Array(array=w437, index=w436) -> (element=w431:string)
            n258 = call-poly <vilib>:"Write Key.vi"("section"=w442, "value"=w431, "key"="Size", "refnum"=w427) -> ("refnum out"=w444:T17)  [unwired: 2 in, 5 out]
            n259 = call-poly <vilib>:"Write Key.vi"("section"=w442, "value"=w433, "key"="FrameRate", "refnum"=w444) -> ("refnum out"=w443:T17)  [unwired: 1 in, 6 out]
            n260 = property on="Camera Settings" class="Clust (strict)"("Visible"=w445) -> ()  [unwired: 2 in, 2 out]
            n261 = local write "DB Camera Config"(w445) -> ()
            n262 = call-poly <vilib>:"Write Key.vi"("section"=w442, "value"=w432, "key"="Compression", "refnum"=w443) -> ("refnum out"=w429:T17)  [unwired: 1 in, 6 out]
            n263 = call <vilib>:"Close Config Data.vi"("refnum"=w429) -> ("file path"=w430:path)  [unwired: 2 in, 8 out]
            n264 = call <vilib>:"Open Config Data.vi"("configuration file path"=w430) -> ("refnum"=w428:T17)  [unwired: 8 in, 2 out]
          }
          frame True {
            n265 = property on="Camera Settings" class="Clust (strict)"("Visible"=TRUE) -> ()  [unwired: 2 in, 2 out]
          }
        }
      }
      event "Camera Settings": Value Change {
        n266 = event-data() -> ("NewVal"=w459:T2)  [unwired: 1 in]
        n267 = Index Array(array=w455) -> (element=w454:cluster{string[]})  [unwired: 1 in]
        n268 = Unbundle(w459) -> ("Frame Rate"=w450:i32, "Compression"=w449:i32, "Size"=w452:u16)
        n269 = Unbundle(w454) -> (w453:string[])
        n270 = Index Array(array=w453, index=w452) -> (element=w451:string)
        n271 = Format Into String(format string="%s   %dfps   %d%%", w451, w450, w449) -> (resulting string=w456:string)  [unwired: 2 in, 1 out]
        n272 = Build Array(w456) -> (w457:string[])
        n273 = property on="DB Camera Config" class="Bool (strict)"("Strings [4]"=w457) -> ()  [unwired: 2 in, 2 out]
      }
      event "Motor.Enable": Value Change {
        n274 = event-data() -> ("NewVal"=w465:bool)  [unwired: 1 in]
        n275 = Unbundle("Motor") -> ("Value"=w464:dbl)  [unwired: 1 out]
        n276 = Select(t=w464, s=w465, f=0.0) -> (s? t:f=w462:dbl)
        n277 = call <vilib>:"NT Write Number.vi"("Numeric"=w462, "Name"=w461) -> ()  [unwired: 9 in, 1 out]
      }
      event "Test Slider": Value Change {
        n278 = event-data() -> ("NewVal"=w468:dbl)  [unwired: 1 in]
        n279 = call <vilib>:"NT Write Number.vi"("Numeric"=w468, "Name"=w469) -> ()  [unwired: 9 in, 1 out]
      }
      event "On/Off": Value Change {
        n280 = event-data() -> ("NewVal"=w473:bool)  [unwired: 1 in]
        n281 = Boolean To (0,1)(Boolean=w473) -> (0, 1=w472:i16)
        n282 = call <vilib>:"NT Write Number.vi"("Numeric"=w472, "Name"=w471) -> ()  [unwired: 9 in, 1 out]
      }
      event "Rev/Fwd": Value Change {
        n283 = event-data() -> ("NewVal.Forward"=w481:bool, "NewVal.Reverse"=w480:bool)  [unwired: 1 in]
        n284 = Boolean To (0,1)(Boolean=w481) -> (0, 1=w477:i16)
        n285 = Boolean To (0,1)(Boolean=w480) -> (0, 1=w479:i16)
        n286 = Negate(x=w479) -> (-x=w478:i16)
        n287 = Add(x=w477, y=w478) -> (x+y=w476:i16)
        n288 = call <vilib>:"NT Write Number.vi"("Numeric"=w476, "Name"=w475) -> ()  [unwired: 9 in, 1 out]
      }
      event "Test Ring": Value Change {
        n289 = event-data() -> ("NewVal"=w485:u16)  [unwired: 1 in]
        n290 = property on="Test Ring" class="Ring (strict)"() -> ("Strings []"=w486:string[])  [unwired: 2 in, 2 out]
        n291 = Index Array(array=w486, index=w485) -> (element=w484:string)
        n292 = call <vilib>:"NT Write String.vi"("String"=w484, "Name"=w483) -> ()  [unwired: 9 in, 1 out]
      }
      event "Rec Mode": Value Change {
        # "Update globals for recording mode and path to read log from.\nClear when logging and let NetworkTables set path for vision to\nuse."
        n293 = event-data() -> ("NewVal"=w496:enum32{"Stop", "Record", "Playback"})  [unwired: 1 in]
        n294 = global write "WPI_DashboardLogging Global.vi" "Logging Filename"(path "") -> ()
        n295 = case shown="\"Stop\", \"Record\"" w496 {
          tunnel: w495 -> [_ w498 w506]
          tunnel: [_ _ w505] -> w492
          tunnel: [_ _ w504] -> _
          tunnel: w490 -> [_ _ w502]
          tunnel: cluster{i32, i32} {-250, 170} -> [_ _ w501]
          tunnel: [_ _ T19 {"Image Size"=TRUE, "Image Type"=TRUE, "Pixel Value"=TRUE, "ROI Information"=TRUE, "Zoom Factor"=FALSE} ("Image Information Shown:All Elements")] -> w488
          tunnel: [_ _ TRUE ("Zoom Factor")] -> w487
          frame Default {
          }
          frame "Stop", "Record" {
            # "Place Window too"
            n296 = invoke class="VI" method="FP.Close"(reference=w498) -> (reference out=w497:refnum<vi>)  [unwired: 2 in, 2 out]
            n297 = invoke class="VI" method="Abort VI"(reference=w497) -> ()  [unwired: 2 in, 3 out]
          }
          frame "Playback" {
            n298 = call "Open Playback Panel.vi"("Offset"=w501, "DB VI Ref"=w502, "Playback in"=w506) -> ("Playback out"=w503:refnum<vi>)  [unwired: 8 in]
            n299 = register-events(w503) -> (reference out=w505:refnum<event-registration>, error out=w504:errorcluster)  [unwired: 2 in]
          }
        }
        n300 = global write "WPI_DashboardLogging Global.vi" "Recording"(w496) -> ()
        n301 = property on="Camera Image" class="ImageControl"("Image Information Shown"=w488, "Image Information Visible"=w487) -> ()  [unwired: 2 in, 2 out]
        n302 = call <vilib>:"WPI_DashboardNT Log FieldName Cache.vi"("Operation"=enum16{"Lookup/Add", "Index", "Clear"}."Clear") -> ()  [unwired: 8 in, 3 out]
      }
      event Panel Close {
        w507 = enum32{"Stop", "Record", "Playback"}."Stop" ("Rec Mode")
        n303 = event-data() -> ()  [unwired: 1 in, 4 out]
        n304 = local write "Rec Mode"(w507) -> ()
        n305 = global write "WPI_DashboardLogging Global.vi" "Recording"(w507) -> ()
      }
      event Panel Close {
        # "Abort playback window and ourself"
        n306 = event-data() -> ()  [unwired: 1 in, 4 out]
        n307 = invoke class="VI" method="FP.Close"(reference=w512) -> (reference out=w511:refnum<vi>)  [unwired: 2 in, 2 out]
        n308 = invoke class="VI" method="Abort VI"(reference=w511) -> (error out=w510:errorcluster)  [unwired: 2 in, 2 out]
        n309 = invoke class="VI" method="Abort VI"(error in=w510) -> ()  [unwired: 2 in, 3 out]
      }
    }
  }
  n310 = property on="On/Off" class="Bool (strict)"("Visible"=w55) -> ()  [unwired: 2 in, 2 out]
  n311 = property on="Motor" class="Clust (strict)"("Visible"=w55) -> ()  [unwired: 2 in, 2 out]
  n312 = property on="Progress" class="Clust (strict)"("Visible"=w55) -> ()  [unwired: 2 in, 2 out]
  n313 = property on="Test Ring" class="Ring (strict)"("Visible"=w55) -> ()  [unwired: 2 in, 2 out]
  n314 = property on="Rev/Fwd" class="Clust (strict)"("Visible"=w55) -> ()  [unwired: 2 in, 2 out]
  n315 = property on="Camera Settings" class="Clust (strict)"("Visible"=w55) -> ()  [unwired: 2 in, 2 out]
  n316 = local write "DB Camera Config"(w55) -> ()
  n317 = global write "WPI_DashboardLogging Global.vi" "Recording"(w38) -> ()
  n318 = local write "Rec Mode"(w38) -> ()
